vi "Problem1-Recevier.vi"() -> ()   [LabVIEW 2017]
panel:
  out "Z":dbl
  out "Y":dbl
  out "X":dbl
  in  "stop":bool
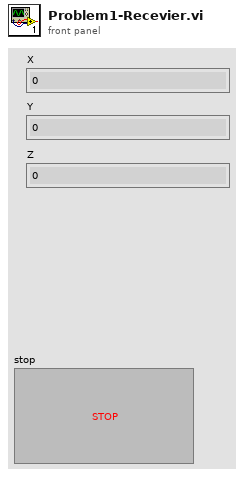
[diagram p1: front panel]
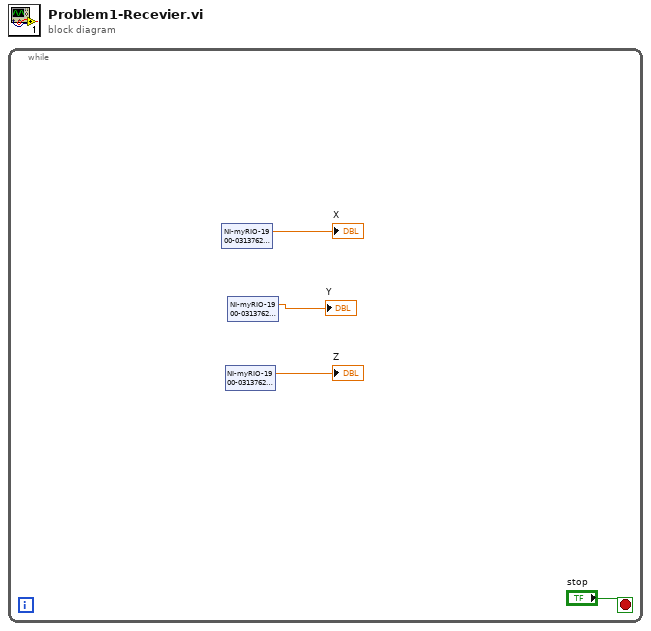
[diagram p0: block diagram]
diagram:
  n1 = while {
    stop <- "stop" stop-if-true
    n2 = shared-variable "NI-myRIO-1900-03137620\\sharedVaraible.lvlib\\x"() -> (→"X":dbl)  [unwired: 1 in, 1 out]
    n3 = shared-variable "NI-myRIO-1900-03137620\\sharedVaraible.lvlib\\z"() -> (→"Z":dbl)  [unwired: 1 in, 1 out]
    n4 = shared-variable "NI-myRIO-1900-03137620\\sharedVaraible.lvlib\\y"() -> (→"Y":dbl)  [unwired: 1 in, 1 out]
  }
